vi "mqtt deregister user events.vi"(1 "Event Registration Refnum in":refnum<event-registration>) -> ()   [LabVIEW 2017]
uses:
  mqtt-LabVIEW/src/class/mqtt/mqttTXqueue/mqttRXsubscriptionEventData.ctl
  mqtt-LabVIEW/src/class/mqtt/mqttTXqueue/mqttTXdataQueueFunction.ctl
  mqtt-LabVIEW/src/class/mqtt/mqttTXqueue/mqttRXsubscriptionEventFunction.ctl
  mqtt-LabVIEW/src/class/mqtt/mqtt.lvclass
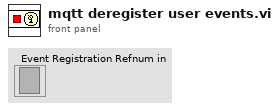
[diagram p1: front panel]
types:
  T1 = typedef "mqttRXsubscriptionEventFunction.ctl" = enum16{"init", "deinit", "getEventRef", "event"}
  T2 = typedef "mqttTXdataQueueFunction.ctl" = enum16{"init", "deinit", "getQueue", "enqueue"}
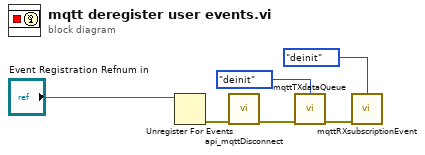
[diagram p0: block diagram]
diagram:
  n1 = Unregister For Events(event registration refnum="Event Registration Refnum in") -> (error out=w5:errorcluster)  [unwired: 1 in]
  n2 = call "api_mqttDisconnect.vi"("error in (no error)"=w5) -> ("error out"=w2:errorcluster)  [unwired: 13 in, 1 out]
  n3 = call "mqttTXdataQueue.vi"("function"=mqttTXdataQueueFunction."deinit", "error in (no error)"=w2) -> ("error out"=w4:errorcluster)  [unwired: 12 in, 1 out]
  n4 = call "mqttRXsubscriptionEvent.vi"("function"=mqttRXsubscriptionEventFunction."deinit", "error in (no error)"=w4) -> ()  [unwired: 12 in, 2 out]
